vi "ConfigTiming.vi"(0 "Task in":refnum<class "WaveformTask.lvclass">, 1 "Sample Mode":enum16{"Finite Samples", "Continuous Samples"}(ring), 3 "Samples per Channel":i32=1000, 9 "Sample Rate":u32=1000, 11 "error in (no error)":errorcluster) -> (4 "Task out":refnum<class "WaveformTask.lvclass">, 10 "Buffer Size [Total Samples]":u32=500000, 15 "error out":errorcluster)   [LabVIEW 2017, in "WaveformTask.lvclass"]
uses:
  WaveformTask.lvclass
  WaveformTask.lvclass/WaveformTask.ctl
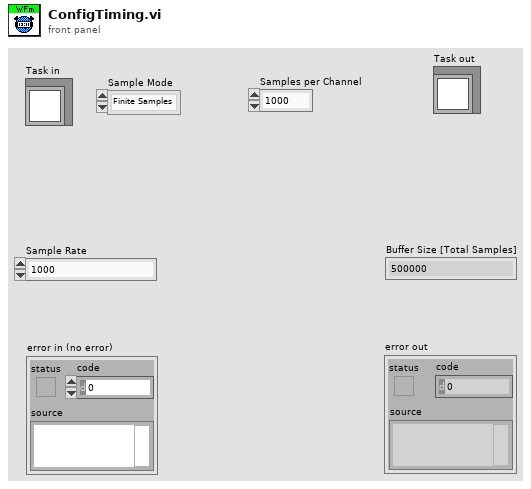
[diagram p1: front panel]
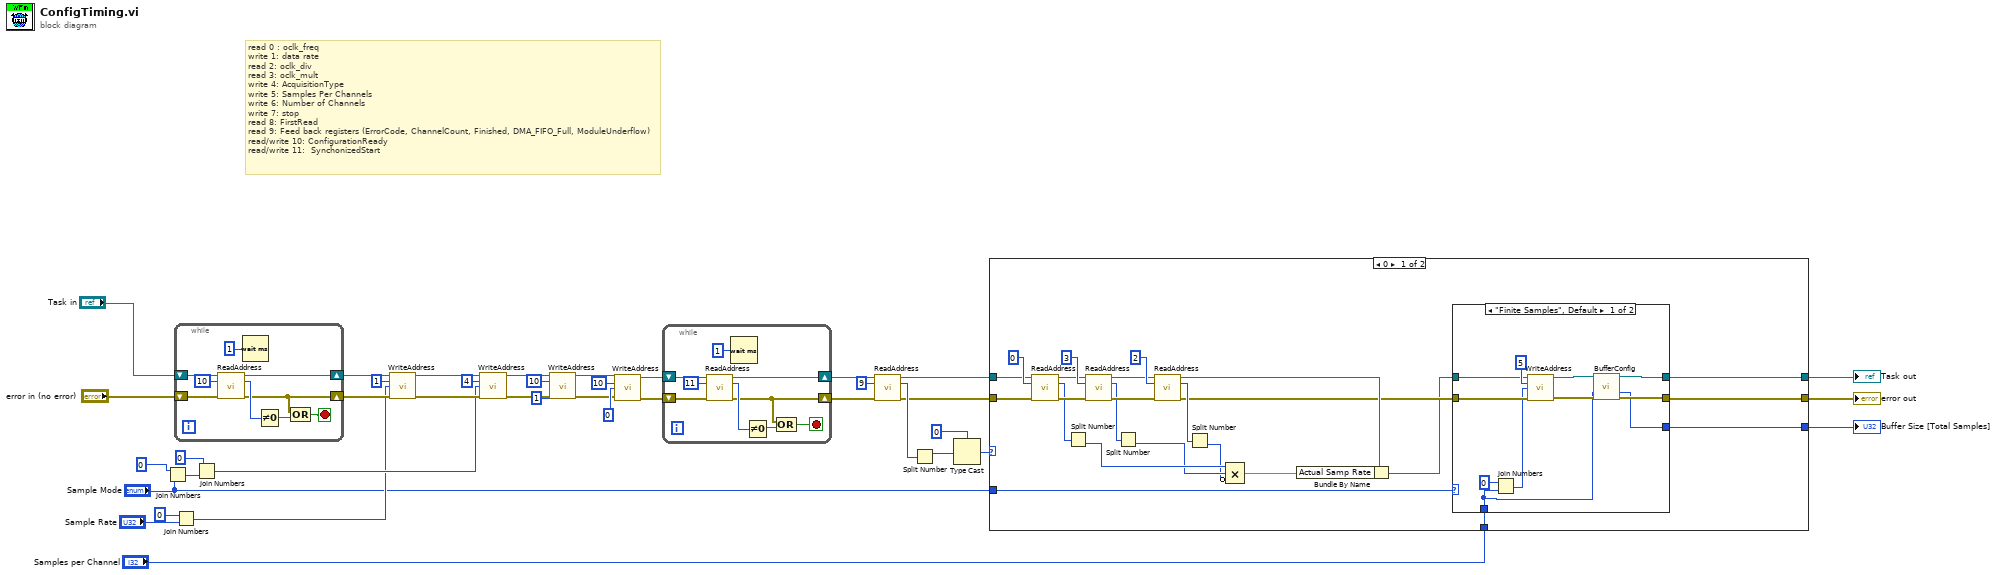
[diagram p0: block diagram]
diagram:
  # "read 0 : oclk_freq\nwrite 1: data rate\nread 2: oclk_div\nread 3: oclk_mult\nwrite 4: AcquisitionType\nwrite 5: Samples Per Channels\nwrite 6: Number of Channels\nwrite 7: stop\nread 8: FirstRead\nread 9: Feed back registers (ErrorCode, ChannelCount, Finished, DMA_FIFO_Full, ModuleUnderflow)\nread/write 10: ConfigurationReady\nread/write 11:  SynchonizedStart"
  n1 = Join Numbers(hi=u16 0, lo="Sample Mode") -> ((hi.lo)=w31:u32)
  n2 = Join Numbers(hi=u32 0, lo="Sample Rate") -> ((hi.lo)=w26:u64)
  n3 = while {
    shift-right: [w47] -> w37
    shift-left: "Task in" -> [w48]
    shift-right: [w41] -> w36
    shift-left: "error in (no error)" -> [w46]
    stop <- w40 stop-if-true
    n4 = call "ReadAddress.vi"("Task in"=w48, "address"=u64 10, "error in (no error)"=w46) -> ("Task out"=w47:refnum<class "WaveformTask.lvclass">, "data"=w44:u64, "error out"=w41:errorcluster)  [unwired: 10 in]
    n5 = Wait (ms)(milliseconds to wait=u32 1) -> ()  [unwired: 1 out]
    n6 = Not Equal To 0?(x=w44) -> (x != 0?=w42:bool)
    n7 = Compound Arithmetic op=OR(w41, w42) -> (w40:bool)
  }
  n8 = Join Numbers(hi=u32 0, lo=w31) -> ((hi.lo)=w29:u64)
  n9 = call "WriteAddress.vi"("Task in"=w37, "address"=u64 1, "data"=w26, "error in (no error)"=w36) -> ("Task out"=w35:refnum<class "WaveformTask.lvclass">, "error out"=w34:errorcluster)  [unwired: 10 in]
  n10 = call "WriteAddress.vi"("Task in"=w35, "address"=u64 4, "data"=w29, "error in (no error)"=w34) -> ("Task out"=w23:refnum<class "WaveformTask.lvclass">, "error out"=w24:errorcluster)  [unwired: 10 in]
  n11 = call "WriteAddress.vi"("Task in"=w23, "address"=u64 10, "data"=u64 1, "error in (no error)"=w24) -> ("Task out"=w18:refnum<class "WaveformTask.lvclass">, "error out"=w17:errorcluster)  [unwired: 10 in]
  n12 = call "WriteAddress.vi"("Task in"=w18, "address"=u64 10, "data"=u64 0, "error in (no error)"=w17) -> ("Task out"=w16:refnum<class "WaveformTask.lvclass">, "error out"=w15:errorcluster)  [unwired: 10 in]
  n13 = while {
    shift-right: [w56] -> w14
    shift-left: w16 -> [w57]
    shift-right: [w50] -> w13
    shift-left: w15 -> [w55]
    stop <- w49 stop-if-true
    n14 = call "ReadAddress.vi"("Task in"=w57, "address"=u64 11, "error in (no error)"=w55) -> ("Task out"=w56:refnum<class "WaveformTask.lvclass">, "data"=w53:u64, "error out"=w50:errorcluster)  [unwired: 10 in]
    n15 = Wait (ms)(milliseconds to wait=u32 1) -> ()  [unwired: 1 out]
    n16 = Not Equal To 0?(x=w53) -> (x != 0?=w51:bool)
    n17 = Compound Arithmetic op=OR(w50, w51) -> (w49:bool)
  }
  n18 = call "ReadAddress.vi"("Task in"=w14, "address"=u64 9, "error in (no error)"=w13) -> ("Task out"=w7:refnum<class "WaveformTask.lvclass">, "data"=w11:u64, "error out"=w6:errorcluster)  [unwired: 10 in]
  n19 = Split Number(x=w11) -> (hi(x)=w10:u32)  [unwired: 1 out]
  n20 = Type Cast(type=0, x=w10) -> (*(type *) &x=w8:i32)
  n21 = case shown="0" w8 {
    tunnel: w7 -> [w80 w96]
    tunnel: w6 -> [w79 w95]
    tunnel: "Sample Mode" -> [w65 _]
    tunnel: [w62 w96] -> w4
    tunnel: [w61 w95] -> w3
    tunnel: "Samples per Channel" -> [w59 _]
    tunnel: [w58 _] -> w1
    frame 0 {
      n22 = call "ReadAddress.vi"("Task in"=w80, "address"=u64 0, "error in (no error)"=w79) -> ("Task out"=w77:refnum<class "WaveformTask.lvclass">, "data"=w72:u64, "error out"=w76:errorcluster)  [unwired: 10 in]
      n23 = Split Number(x=w72) -> (lo(x)=w69:u32)  [unwired: 1 out]
      n24 = call "ReadAddress.vi"("Task in"=w77, "address"=u64 3, "error in (no error)"=w76) -> ("Task out"=w74:refnum<class "WaveformTask.lvclass">, "data"=w71:u64, "error out"=w73:errorcluster)  [unwired: 10 in]
      n25 = Split Number(x=w71) -> (lo(x)=w68:u32)  [unwired: 1 out]
      n26 = call "ReadAddress.vi"("Task in"=w74, "address"=u64 2, "error in (no error)"=w73) -> ("Task out"=w64:refnum<class "WaveformTask.lvclass">, "data"=w70:u64, "error out"=w63:errorcluster)  [unwired: 10 in]
      n27 = Split Number(x=w70) -> (lo(x)=w67:u32)  [unwired: 1 out]
      n28 = Compound Arithmetic op=MULTIPLY(w69, w68, invert w67) -> (w66:dbl)
      n29 = Bundle By Name(cluster=w64, "Actual Samp Rate"=w66) -> (w60:refnum<class "WaveformTask.lvclass">)
      n30 = case shown="\"Finite Samples\", Default" w65 {
        tunnel: w60 -> [w91 w94]
        tunnel: w63 -> [w90 w93]
        tunnel: [w84 w94] -> w62
        tunnel: [w83 w93] -> w61
        tunnel: w59 -> [w85 _]
        tunnel: [w82 _] -> w58
        frame "Finite Samples", Default {
          n31 = Join Numbers(hi=0, lo=w85) -> ((hi.lo)=w88:u64)
          n32 = call "WriteAddress.vi"("Task in"=w91, "address"=u64 5, "data"=w88, "error in (no error)"=w90) -> ("Task out"=w87:refnum<class "WaveformTask.lvclass">, "error out"=w86:errorcluster)  [unwired: 10 in]
          n33 = call "BufferConfig.vi"("WaveformTask in"=w87, "Buffer Size [Samps per Chan]"=w85, "error in (no error)"=w86) -> ("WaveformTask out"=w84:refnum<class "WaveformTask.lvclass">, "Buffer Size [Total Samples]"=w82:u32, "error out"=w83:errorcluster)  [unwired: 10 in]
        }
        frame "Continuous Samples" {
        }
      }
    }
    frame Default {
    }
  }
  "Task out" <- w4
  "error out" <- w3
  "Buffer Size [Total Samples]" <- w1
